vi "LIN_LDF_Load.vi"(7 "DataBase_array":T1, 8 "error in (no error)":errorcluster caption="错误输入（无错误）", 9 "Channels":i32[](array[numeric]), 10 "LDF Path":path, 11 "DLL_PATH":path) -> (0 "error out":errorcluster caption="错误输出", 3 "result":bool)   [LabVIEW 2014]
uses:
  Typedef/CAN/TCANSignal.ctl
  Typedef/LIN/TLINSignal.ctl
  Typedef/FlexRay/TFlexRaySignal.ctl
  Typedef/TDBSignalProperties.ctl
  Typedef/TDBFrameProperties.ctl
  Typedef/TDBECUProperties.ctl
  Typedef/TDBProperties.ctl
  Typedef/DataBase_array.ctl
  Typedef/DataBase_array_index.ctl
types:
  T1 = typedef "DataBase_array_index.ctl" = refnum<vi>
  T2 = typedef "TDBProperties.ctl" = cluster{"FDBIndex":i32, "FSignalCount":i32, "FFrameCount":i32, "FECUCount":i32, "FSupportedChannelMask":u64, "FName":cluster{"数值":u64, "数值 2":u64, "数值 3":u64, "数值 4":u64, "数值 5":u64, "数值 6":u64, "数值 7":u64, "数值 8":u64, "数值 9":u64, "数值 10":u64, "数值 11":u64, "数值 12":u64, "数值 13":u64, "数值 14":u64, "数值 15":u64, "数值 16":u64, "数值 17":u64, "数值 18":u64, "数值 19":u64, "数值 20":u64, "数值 21":u64, "数值 22":u64, "数值 23":u64, "数值 24":u64, "数值 25":u64, "数值 26":u64, "数值 27":u64, "数值 28":u64, "数值 29":u64, "数值 30":u64, "数值 31":u64, "数值 32":u64, "数值 33":u64, "数值 34":u64, "数值 35":u64, "数值 36":u64, "数值 37":u64, "数值 38":u64, "数值 39":u64, "数值 40":u64, "数值 41":u64, "数值 42":u64, "数值 43":u64, "数值 44":u64, "数值 45":u64, "数值 46":u64, "数值 47":u64, "数值 48":u64, "数值 49":u64, "数值 50":u64, "数值 51":u64, "数值 52":u64, "数值 53":u64, "数值 54":u64, "数值 55":u64, "数值 56":u64, "数值 57":u64, "数值 58":u64, "数值 59":u64, "数值 60":u64, "数值 61":u64, "数值 62":u64, "数值 63":u64, "数值 64":u64}, "FComment":cluster{"数值":u64, "数值 2":u64, "数值 3":u64, "数值 4":u64, "数值 5":u64, "数值 6":u64, "数值 7":u64, "数值 8":u64, "数值 9":u64, "数值 10":u64, "数值 11":u64, "数值 12":u64, "数值 13":u64, "数值 14":u64, "数值 15":u64, "数值 16":u64, "数值 17":u64, "数值 18":u64, "数值 19":u64, "数值 20":u64, "数值 21":u64, "数值 22":u64, "数值 23":u64, "数值 24":u64, "数值 25":u64, "数值 26":u64, "数值 27":u64, "数值 28":u64, "数值 29":u64, "数值 30":u64, "数值 31":u64, "数值 32":u64, "数值 33":u64, "数值 34":u64, "数值 35":u64, "数值 36":u64, "数值 37":u64, "数值 38":u64, "数值 39":u64, "数值 40":u64, "数值 41":u64, "数值 42":u64, "数值 43":u64, "数值 44":u64, "数值 45":u64, "数值 46":u64, "数值 47":u64, "数值 48":u64, "数值 49":u64, "数值 50":u64, "数值 51":u64, "数值 52":u64, "数值 53":u64, "数值 54":u64, "数值 55":u64, "数值 56":u64, "数值 57":u64, "数值 58":u64, "数值 59":u64, "数值 60":u64, "数值 61":u64, "数值 62":u64, "数值 63":u64, "数值 64":u64}, "FFlags":u32, "FDBId":u32}
  T3 = typedef "TDBECUProperties.ctl" = cluster{"FDBIndex":i32, "FECUIndex":i32, "FTxFrameCount":i32, "FRxFrameCount":i32, "FName":cluster{"数值":u64, "数值 2":u64, "数值 3":u64, "数值 4":u64, "数值 5":u64, "数值 6":u64, "数值 7":u64, "数值 8":u64, "数值 9":u64, "数值 10":u64, "数值 11":u64, "数值 12":u64, "数值 13":u64, "数值 14":u64, "数值 15":u64, "数值 16":u64, "数值 17":u64, "数值 18":u64, "数值 19":u64, "数值 20":u64, "数值 21":u64, "数值 22":u64, "数值 23":u64, "数值 24":u64, "数值 25":u64, "数值 26":u64, "数值 27":u64, "数值 28":u64, "数值 29":u64, "数值 30":u64, "数值 31":u64, "数值 32":u64, "数值 33":u64, "数值 34":u64, "数值 35":u64, "数值 36":u64, "数值 37":u64, "数值 38":u64, "数值 39":u64, "数值 40":u64, "数值 41":u64, "数值 42":u64, "数值 43":u64, "数值 44":u64, "数值 45":u64, "数值 46":u64, "数值 47":u64, "数值 48":u64, "数值 49":u64, "数值 50":u64, "数值 51":u64, "数值 52":u64, "数值 53":u64, "数值 54":u64, "数值 55":u64, "数值 56":u64, "数值 57":u64, "数值 58":u64, "数值 59":u64, "数值 60":u64, "数值 61":u64, "数值 62":u64, "数值 63":u64, "数值 64":u64}, "FComment":cluster{"数值":u64, "数值 2":u64, "数值 3":u64, "数值 4":u64, "数值 5":u64, "数值 6":u64, "数值 7":u64, "数值 8":u64, "数值 9":u64, "数值 10":u64, "数值 11":u64, "数值 12":u64, "数值 13":u64, "数值 14":u64, "数值 15":u64, "数值 16":u64, "数值 17":u64, "数值 18":u64, "数值 19":u64, "数值 20":u64, "数值 21":u64, "数值 22":u64, "数值 23":u64, "数值 24":u64, "数值 25":u64, "数值 26":u64, "数值 27":u64, "数值 28":u64, "数值 29":u64, "数值 30":u64, "数值 31":u64, "数值 32":u64, "数值 33":u64, "数值 34":u64, "数值 35":u64, "数值 36":u64, "数值 37":u64, "数值 38":u64, "数值 39":u64, "数值 40":u64, "数值 41":u64, "数值 42":u64, "数值 43":u64, "数值 44":u64, "数值 45":u64, "数值 46":u64, "数值 47":u64, "数值 48":u64, "数值 49":u64, "数值 50":u64, "数值 51":u64, "数值 52":u64, "数值 53":u64, "数值 54":u64, "数值 55":u64, "数值 56":u64, "数值 57":u64, "数值 58":u64, "数值 59":u64, "数值 60":u64, "数值 61":u64, "数值 62":u64, "数值 63":u64, "数值 64":u64}}
  T4 = typedef "TDBFrameProperties.ctl" = cluster{"FDBIndex":i32, "FECUIndex":i32, "FFrameIndex":i32, "FIsTx":u8, "FReserved1":u8, "FCycleTimeMs":u16, "TSignalType":i32, "FCANIsDataFrame":u8, "FCANIsStdFrame":u8, "FCANIsEdl":u8, "FCANIsBrs":u8, "FCANIdentifier":i32, "FCANDLC":i32, "FCANDataBytes":i32, "FLINIdentifier":i32, "FLINDLC":i32, "FFRChannelMask":u8, "FFRBaseCycle":u8, "FFRCycleRepetition":u8, "FFRIsStartupFrame":u8, "FFRSlotId":u16, "FFRDLC":u16, "FFRCycleMask":u64, "FSignalCount":i32, "FName":cluster{"数值":u64, "数值 2":u64, "数值 3":u64, "数值 4":u64, "数值 5":u64, "数值 6":u64, "数值 7":u64, "数值 8":u64, "数值 9":u64, "数值 10":u64, "数值 11":u64, "数值 12":u64, "数值 13":u64, "数值 14":u64, "数值 15":u64, "数值 16":u64, "数值 17":u64, "数值 18":u64, "数值 19":u64, "数值 20":u64, "数值 21":u64, "数值 22":u64, "数值 23":u64, "数值 24":u64, "数值 25":u64, "数值 26":u64, "数值 27":u64, "数值 28":u64, "数值 29":u64, "数值 30":u64, "数值 31":u64, "数值 32":u64, "数值 33":u64, "数值 34":u64, "数值 35":u64, "数值 36":u64, "数值 37":u64, "数值 38":u64, "数值 39":u64, "数值 40":u64, "数值 41":u64, "数值 42":u64, "数值 43":u64, "数值 44":u64, "数值 45":u64, "数值 46":u64, "数值 47":u64, "数值 48":u64, "数值 49":u64, "数值 50":u64, "数值 51":u64, "数值 52":u64, "数值 53":u64, "数值 54":u64, "数值 55":u64, "数值 56":u64, "数值 57":u64, "数值 58":u64, "数值 59":u64, "数值 60":u64, "数值 61":u64, "数值 62":u64, "数值 63":u64, "数值 64":u64}, "FComment":cluster{"数值":u64, "数值 2":u64, "数值 3":u64, "数值 4":u64, "数值 5":u64, "数值 6":u64, "数值 7":u64, "数值 8":u64, "数值 9":u64, "数值 10":u64, "数值 11":u64, "数值 12":u64, "数值 13":u64, "数值 14":u64, "数值 15":u64, "数值 16":u64, "数值 17":u64, "数值 18":u64, "数值 19":u64, "数值 20":u64, "数值 21":u64, "数值 22":u64, "数值 23":u64, "数值 24":u64, "数值 25":u64, "数值 26":u64, "数值 27":u64, "数值 28":u64, "数值 29":u64, "数值 30":u64, "数值 31":u64, "数值 32":u64, "数值 33":u64, "数值 34":u64, "数值 35":u64, "数值 36":u64, "数值 37":u64, "数值 38":u64, "数值 39":u64, "数值 40":u64, "数值 41":u64, "数值 42":u64, "数值 43":u64, "数值 44":u64, "数值 45":u64, "数值 46":u64, "数值 47":u64, "数值 48":u64, "数值 49":u64, "数值 50":u64, "数值 51":u64, "数值 52":u64, "数值 53":u64, "数值 54":u64, "数值 55":u64, "数值 56":u64, "数值 57":u64, "数值 58":u64, "数值 59":u64, "数值 60":u64, "数值 61":u64, "数值 62":u64, "数值 63":u64, "数值 64":u64}}
  T5 = typedef "TDBSignalProperties.ctl" = cluster{"FDBIndex":i32, "FECUIndex":i32, "FFrameIndex":i32, "FSignalIndex":i32, "FIsTx":u8, "FReserved1":u8, "FReserved2":u8, "FReserved3":u8, "TSignalType":i32, "TCANSignal":T6, "TLINSignal":T7, "TFlexRaySignal":T8, "FParentFrameId":i32, "FInitValue":dbl, "FName":cluster{"数值":u64, "数值 2":u64, "数值 3":u64, "数值 4":u64, "数值 5":u64, "数值 6":u64, "数值 7":u64, "数值 8":u64, "数值 9":u64, "数值 10":u64, "数值 11":u64, "数值 12":u64, "数值 13":u64, "数值 14":u64, "数值 15":u64, "数值 16":u64, "数值 17":u64, "数值 18":u64, "数值 19":u64, "数值 20":u64, "数值 21":u64, "数值 22":u64, "数值 23":u64, "数值 24":u64, "数值 25":u64, "数值 26":u64, "数值 27":u64, "数值 28":u64, "数值 29":u64, "数值 30":u64, "数值 31":u64, "数值 32":u64, "数值 33":u64, "数值 34":u64, "数值 35":u64, "数值 36":u64, "数值 37":u64, "数值 38":u64, "数值 39":u64, "数值 40":u64, "数值 41":u64, "数值 42":u64, "数值 43":u64, "数值 44":u64, "数值 45":u64, "数值 46":u64, "数值 47":u64, "数值 48":u64, "数值 49":u64, "数值 50":u64, "数值 51":u64, "数值 52":u64, "数值 53":u64, "数值 54":u64, "数值 55":u64, "数值 56":u64, "数值 57":u64, "数值 58":u64, "数值 59":u64, "数值 60":u64, "数值 61":u64, "数值 62":u64, "数值 63":u64, "数值 64":u64}, "FComment":cluster{"数值":u64, "数值 2":u64, "数值 3":u64, "数值 4":u64, "数值 5":u64, "数值 6":u64, "数值 7":u64, "数值 8":u64, "数值 9":u64, "数值 10":u64, "数值 11":u64, "数值 12":u64, "数值 13":u64, "数值 14":u64, "数值 15":u64, "数值 16":u64, "数值 17":u64, "数值 18":u64, "数值 19":u64, "数值 20":u64, "数值 21":u64, "数值 22":u64, "数值 23":u64, "数值 24":u64, "数值 25":u64, "数值 26":u64, "数值 27":u64, "数值 28":u64, "数值 29":u64, "数值 30":u64, "数值 31":u64, "数值 32":u64, "数值 33":u64, "数值 34":u64, "数值 35":u64, "数值 36":u64, "数值 37":u64, "数值 38":u64, "数值 39":u64, "数值 40":u64, "数值 41":u64, "数值 42":u64, "数值 43":u64, "数值 44":u64, "数值 45":u64, "数值 46":u64, "数值 47":u64, "数值 48":u64, "数值 49":u64, "数值 50":u64, "数值 51":u64, "数值 52":u64, "数值 53":u64, "数值 54":u64, "数值 55":u64, "数值 56":u64, "数值 57":u64, "数值 58":u64, "数值 59":u64, "数值 60":u64, "数值 61":u64, "数值 62":u64, "数值 63":u64, "数值 64":u64}}
  T6 = typedef "TCANSignal.ctl" = cluster{"FCANSgnType":u8, "FIsIntel":u8, "FStartBit":i32, "FLength":i32, "FFactor":dbl, "FOffset":dbl}
  T7 = typedef "TLINSignal.ctl" = cluster{"FLINSgnType":u8, "FIsIntel":u8, "FStartBit":i32, "FLength":i32, "FFactor":dbl, "FOffset":dbl}
  T8 = typedef "TFlexRaySignal.ctl" = cluster{"FFRSgnType":u8, "FCompuMethod":u8, "FReserved":u8, "FIsIntel":u8, "FStartBit":i32, "FUpdateBit":i32, "FLength":i32, "FFactor":dbl, "FOffset":dbl, "FActualStartBit":i32, "FActualUpdateBit":i32}
  T9 = cluster{"TDBECUProperties":T3, cluster{"TDBFrameProperties":T4, T5[]}[], cluster{"TDBFrameProperties":T4, T5[]}[]}
  T10 = cluster{"db_properties":T2, cluster{"TDBECUProperties":T3, cluster{"TDBFrameProperties":T4, T5[]}[], cluster{"TDBFrameProperties":T4, T5[]}[]}[]}
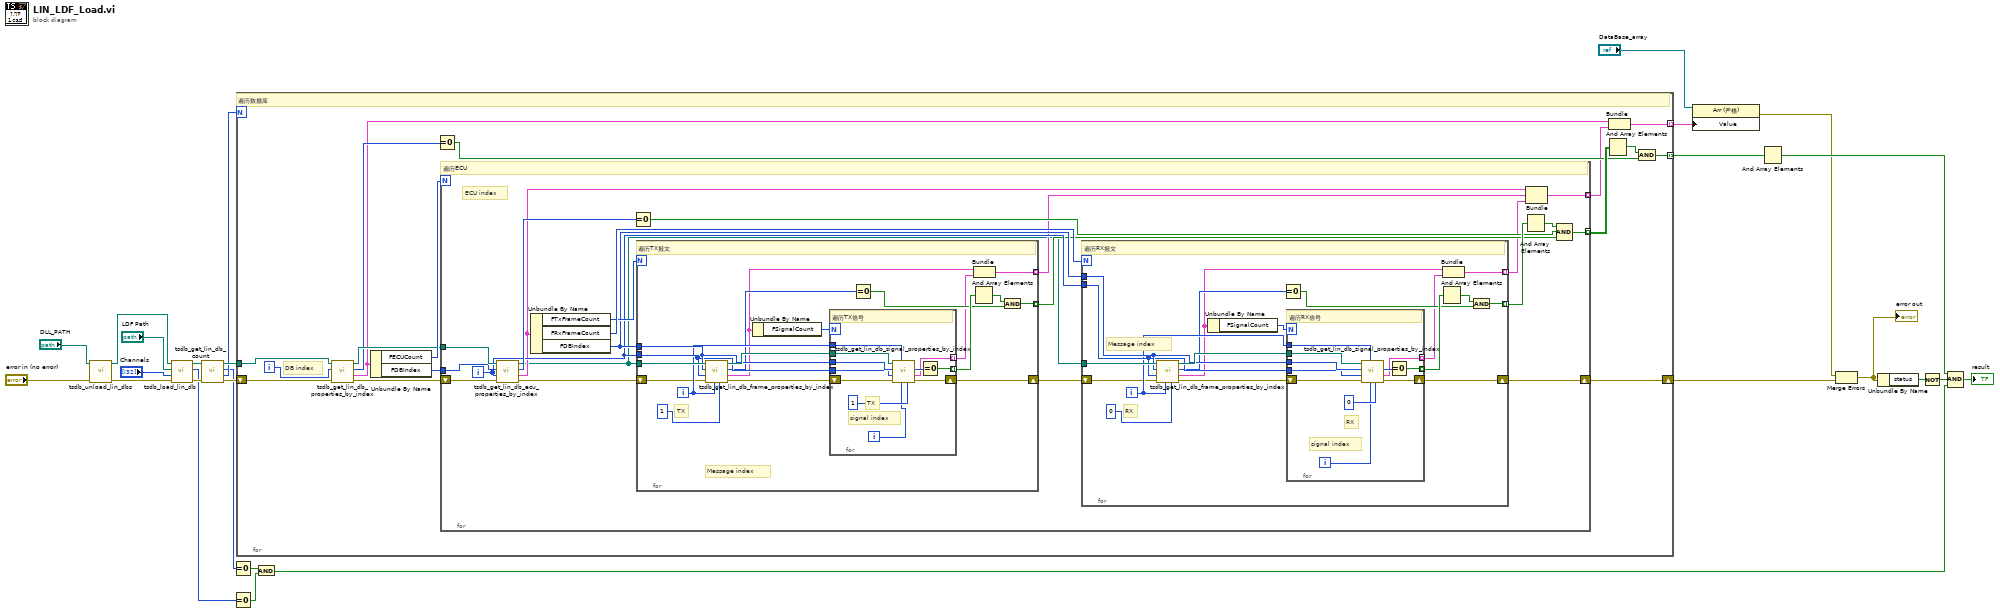
[diagram p0: block diagram]
diagram:
  n1 = call "tsdb_unload_lin_dbs.vi"("error in (no error)"="error in (no error)", "路径输入"="DLL_PATH") -> ("error out"=w23:errorcluster, "路径输出"=w22:path)  [unwired: 7 in, 1 out]
  n2 = call "tsdb_load_lin_db.vi"("error in (no error)"=w23, "ABindChannels"="Channels", "ADBCAbsolutePath"="LDF Path", "路径输入"=w22) -> ("error out"=w25:errorcluster, "function return"=w11:i32, "路径输出"=w24:path)  [unwired: 4 in, 1 out]
  n3 = call "tsdb_get_lin_db_count.vi"("error in (no error)"=w25, "路径输入"=w24) -> ("error out"=w14:errorcluster, "ACount out"=w12:i32, "return"=w10:i32, "路径输出"=w15:path)  [unwired: 6 in]
  n4 = Equal To 0?(x=w10) -> (x = 0?=w8:bool)
  n5 = Equal To 0?(x=w11) -> (x = 0?=w7:bool)
  n6 = for {
    N: w12 -> [_]
    tunnel: w15 -> [w42]
    shift-right: [w35] -> w13
    shift-left: w14 -> [w41]
    tunnel: [w30] -> w9 mode=indexing
    tunnel: [w27] -> w2 mode=indexing
    i -> [w36]
    # "DB index"
    # "遍历数据库"
    n7 = call "tsdb_get_lin_db_properties_by_index.vi"("error in (no error)"=w41, "FDBIndex"=w36, "path in"=w42) -> ("error out"=w39:errorcluster, "db_properties"=w29:T2, "return"=w34:i32, "path out"=w38:path)  [unwired: 5 in]
    n8 = Unbundle By Name(w29) -> ("FECUCount"=w40:i32, "FDBIndex"=w37:i32)
    n9 = Equal To 0?(x=w34) -> (x = 0?=w31:bool)
    n10 = for {
      N: w40 -> [_]
      tunnel: w38 -> [w62]
      shift-right: [w60] -> w35
      shift-left: w39 -> [w63]
      tunnel: w37 -> [w54]
      tunnel: [w55] -> w32 mode=indexing
      tunnel: [w44] -> w28 mode=indexing
      i -> [w51]
      # "ECU index"
      # "遍历ECU"
      n11 = call "tsdb_get_lin_db_ecu_properties_by_index.vi"("error in (no error)"=w63, "FECUIndex"=w51, "FDBIndex"=w54, "路径输入"=w62) -> ("error out"=w48:errorcluster, "TDBECUProperties"=w47:T3, "function return"=w59:i32, "路径输出"=w43:path)  [unwired: 4 in]
      n12 = Unbundle By Name(w47) -> ("FTxFrameCount"=w53:i32, "FRxFrameCount"=w61:i32, "FDBIndex"=w52:i32)
      n13 = Equal To 0?(x=w59) -> (x = 0?=w56:bool)
      n14 = for {
        N: w53 -> [_]
        tunnel: w43 -> [w81]
        tunnel: w52 -> [w79]
        tunnel: w51 -> [w78]
        tunnel: [w71] -> w50 mode=indexing
        tunnel: [w64] -> w46 mode=indexing
        shift-right: [w66] -> w49
        shift-left: w48 -> [w65]
        i -> [w77]
        # "TX"
        # "Message index"
        # "遍历TX报文"
        n15 = call "tsdb_get_lin_db_frame_properties_by_index.vi"("FIsTx"=u8 1, "FFrameIndex"=w77, "error in (no error)"=w65, "FECUIndex"=w78, "FDBIndex"=w79, "路径输入"=w81) -> ("error out"=w67:errorcluster, "TDBFrameProperties"=w69:T4, "function return"=w75:i32, "路径输出"=w80:path)  [unwired: 2 in]
        n16 = Unbundle By Name(w69) -> ("FSignalCount"=w76:i32)
        n17 = for {
          N: w76 -> [_]
          tunnel: w80 -> [w92]
          tunnel: w79 -> [w91]
          tunnel: w78 -> [w90]
          tunnel: w77 -> [w89]
          tunnel: [w85] -> w74 mode=indexing
          tunnel: [w84] -> w68 mode=indexing
          shift-right: [w82] -> w66
          shift-left: w67 -> [w83]
          i -> [w87]
          # "signal index"
          # "TX"
          # "遍历TX信号"
          n18 = call "tsdb_get_lin_db_signal_properties_by_index.vi"("FIsTx"=u8 1, "FSignalIndex"=w87, "FFrameIndex"=w89, "error in (no error)"=w83, "FECUIndex"=w90, "FDBIndex"=w91, "路径输入"=w92) -> ("error out"=w82:errorcluster, "TDBSignalProperties"=w84:T5, "function return"=w86:i32)  [unwired: 1 in, 1 out]
          n19 = Equal To 0?(x=w86) -> (x = 0?=w85:bool)
        }
        n20 = Equal To 0?(x=w75) -> (x = 0?=w72:bool)
        n21 = And Array Elements(Boolean array=w74) -> (logical AND=w73:bool)
        n22 = Bundle("TDBFrameProperties"=w69, w68) -> (w64:cluster{"TDBFrameProperties":T4, T5[]})  [unwired: 1 in]
        n23 = And(x=w73, y=w72) -> (x .and. y?=w71:bool)
      }
      n24 = for {
        N: w61 -> [_]
        tunnel: w43 -> [w110]
        tunnel: w52 -> [w108]
        tunnel: w51 -> [w107]
        tunnel: [w99] -> w57 mode=indexing
        tunnel: [w93] -> w45 mode=indexing
        shift-right: [w95] -> w60
        shift-left: w49 -> [w94]
        i -> [w106]
        # "RX"
        # "Message index"
        # "遍历RX报文"
        n25 = call "tsdb_get_lin_db_frame_properties_by_index.vi"("FIsTx"=u8 0, "FFrameIndex"=w106, "error in (no error)"=w94, "FECUIndex"=w107, "FDBIndex"=w108, "路径输入"=w110) -> ("error out"=w96:errorcluster, "TDBFrameProperties"=w98:T4, "function return"=w103:i32, "路径输出"=w109:path)  [unwired: 2 in]
        n26 = Unbundle By Name(w98) -> ("FSignalCount"=w105:i32)
        n27 = Equal To 0?(x=w103) -> (x = 0?=w100:bool)
        n28 = for {
          N: w105 -> [_]
          tunnel: w109 -> [w121]
          tunnel: w108 -> [w120]
          tunnel: w107 -> [w119]
          tunnel: w106 -> [w118]
          tunnel: [w114] -> w102 mode=indexing
          tunnel: [w113] -> w97 mode=indexing
          shift-right: [w111] -> w95
          shift-left: w96 -> [w112]
          i -> [w116]
          # "signal index"
          # "RX"
          # "遍历RX信号"
          n29 = call "tsdb_get_lin_db_signal_properties_by_index.vi"("FIsTx"=u8 0, "FSignalIndex"=w116, "FFrameIndex"=w118, "error in (no error)"=w112, "FECUIndex"=w119, "FDBIndex"=w120, "路径输入"=w121) -> ("error out"=w111:errorcluster, "TDBSignalProperties"=w113:T5, "function return"=w115:i32)  [unwired: 1 in, 1 out]
          n30 = Equal To 0?(x=w115) -> (x = 0?=w114:bool)
        }
        n31 = And Array Elements(Boolean array=w102) -> (logical AND=w101:bool)
        n32 = Bundle("TDBFrameProperties"=w98, w97) -> (w93:cluster{"TDBFrameProperties":T4, T5[]})  [unwired: 1 in]
        n33 = And(x=w101, y=w100) -> (x .and. y?=w99:bool)
      }
      n34 = And Array Elements(Boolean array=w57) -> (logical AND=w58:bool)
      n35 = Bundle("TDBECUProperties"=w47, w46, w45) -> (w44:T9)  [unwired: 1 in]
      n36 = Compound Arithmetic op=AND(w58, w56, w50) -> (w55:bool[])
    }
    n37 = And Array Elements(Boolean array=w32) -> (logical AND=w33:bool)
    n38 = Bundle("db_properties"=w29, w28) -> (w27:T10)  [unwired: 1 in]
    n39 = And(x=w33, y=w31) -> (x .and. y?=w30:bool)
  }
  n40 = And(x=w8, y=w7) -> (x .and. y?=w6:bool)
  n41 = property class="Arr (严格)"(reference="DataBase_array", "Value"=w2) -> (error out=w3:errorcluster)  [unwired: 1 in, 1 out]
  n42 = And Array Elements(Boolean array=w9) -> (logical AND=w17:bool)
  n43 = Merge Errors(w3, w13) -> (w4:errorcluster)
  "error out" <- w4
  n44 = Unbundle By Name(w4) -> ("status"=w18:bool)
  n45 = Not(x=w18) -> (.not. x?=w16:bool)
  n46 = Compound Arithmetic op=AND(w17, w16, w6) -> (→"result":bool)
